vi "Read Config File.vi"(8 "error in (no error)":errorcluster, 11 "[C] User Management in":refnum<class "[C] User Management.lvclass">) -> (0 "error out":errorcluster, 3 "[C] User Management out":refnum<class "[C] User Management.lvclass">)   [LabVIEW 2020, in "[C] User Management.lvlib" / "[C] User Management.lvclass"]
uses:
  [C] User Management.lvclass
  [C] User Management.lvclass/[C] User Management.ctl
  <vilib>/Utility/config.llb/NI_LVConfig.lvlib
  <userlib>/_OpenG.lib/variantconfig/variantconfig.llb/openg_variant_configuration_file.lvlib
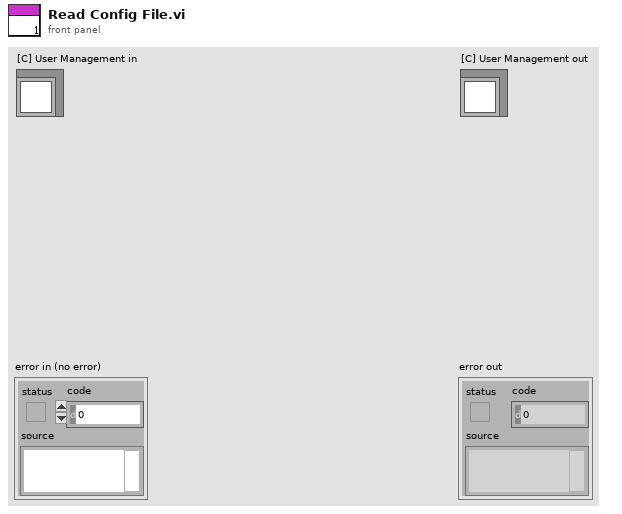
[diagram p1: front panel]
types:
  T1 = cluster{"login":cluster{"enable_rmb_user":bool, "recent_user_list":string[]}}
  T2 = typedef "NI_LVConfig.lvlib/Config Data RefNum.ctl" = refnum<k1>
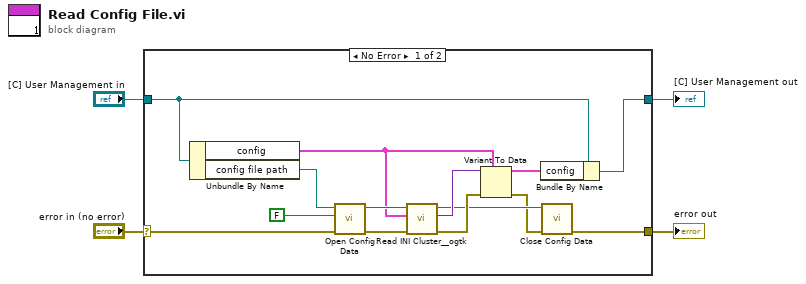
[diagram p0: block diagram]
diagram:
  n1 = case shown="No Error" "error in (no error)" {
    selector: "error in (no error)" -> [w18 w20]
    tunnel: [w5 w20] -> w3
    tunnel: [w6 w19] -> w1
    tunnel: "[C] User Management in" -> [w8 w19]
    frame No Error {
      n2 = Unbundle By Name(w8) -> ("config"=w13:T1, "config file path"=w17:path)
      n3 = call <vilib>:"Open Config Data.vi"("error in (no error)"=w18, "create file if necessary (T)"=FALSE, "configuration file path"=w17) -> ("error out"=w15:errorcluster, "refnum"=w14:T2)  [unwired: 6 in, 1 out]
      n4 = call <userlib>:"Read INI Cluster__ogtk.vi"("error in (no error)"=w15, "INI Fomatted Cluster Type"=w13, "refnum"=w14) -> ("error out"=w11:errorcluster, "INI Fomatted Cluster"=w12:variant, "dup refnum"=w10:T2)  [unwired: 4 in, 2 out]
      n5 = Variant To Data(error in=w11, type=w13, Variant=w12) -> (data=w7:T1, error out=w9:errorcluster)
      n6 = Bundle By Name(cluster=w8, "config"=w7) -> (w6:refnum<class "[C] User Management.lvclass">)
      n7 = call <vilib>:"Close Config Data.vi"("error in (no error)"=w9, "refnum"=w10) -> ("error out"=w5:errorcluster)  [unwired: 8 in, 1 out]
    }
    frame Error {
    }
  }
  "error out" <- w3
  "[C] User Management out" <- w1
